vi "Wirte Fluence Parameter.vi"(8 "#of Areas":i32, 9 "#Overlays":i32, 10 "Size of region (px)":i32, 11 "Analyze Parameter Fluence in":refnum<class "Analyze Parameter Fluence.lvclass">) -> (3 "Analyze Parameter Fluence out":refnum<class "Analyze Parameter Fluence.lvclass">)   [LabVIEW 2014, in "Analyze Parameter Fluence.lvclass"]
uses:
  Analyze Parameter Fluence.lvclass
  Analyze Parameter Fluence.lvclass/Analyze Parameter Fluence.ctl
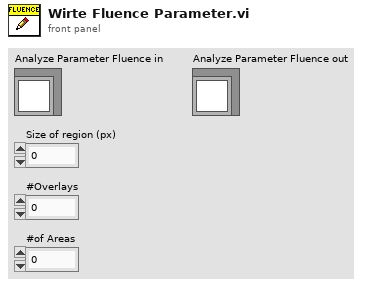
[diagram p1: front panel]
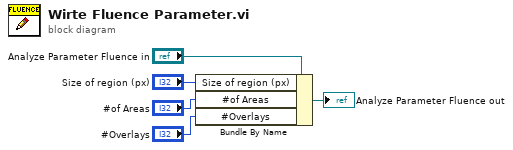
[diagram p0: block diagram]
diagram:
  n1 = Bundle By Name(cluster="Analyze Parameter Fluence in", "Size of region (px)"="Size of region (px)", "#of Areas"="#of Areas", "#Overlays"="#Overlays") -> (→"Analyze Parameter Fluence out":refnum<class "Analyze Parameter Fluence.lvclass">)
